vi "Frequency_list_generation.vi"(8 "Type":enum16{"Logarithmic", "Linear"}(ring)=enum."Linear", 9 "Frequency Points":u16=10 min=2 max=10000 step=1, 10 "Stop Frequency (Hz)":u32(slide)=53143 caption="End Frequency (Hz)" scale=30000.0..100000.0, 11 "Start Frequency (Hz)":u32(slide)=53143 scale=30000.0..100000.0) -> (3 "Frequency List":u32[](array[numeric])=[1000, 1002])   [LabVIEW 2018]
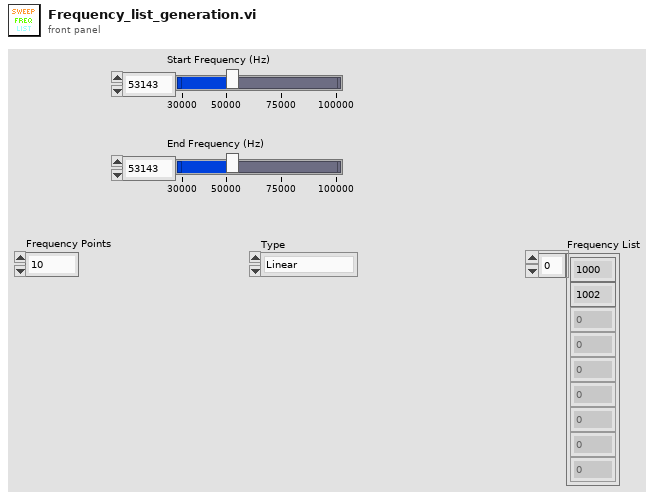
[diagram p1: front panel]
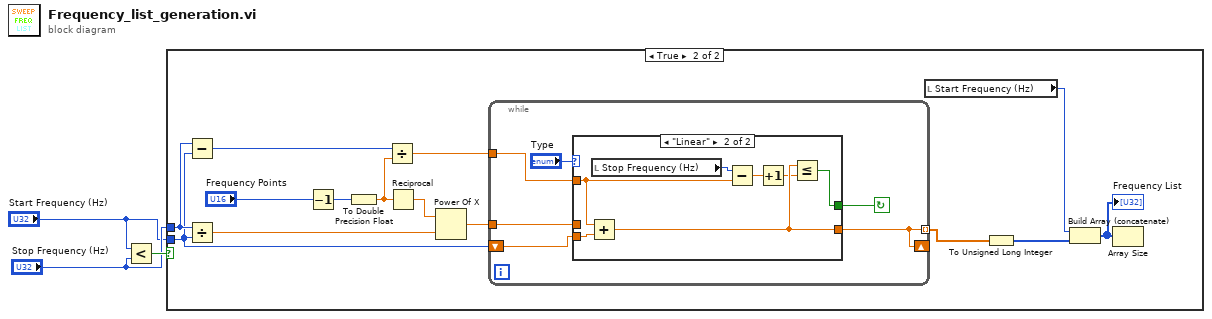
[diagram p0: block diagram]
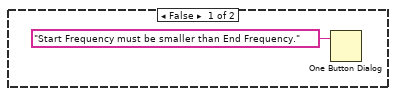
[diagram p2: hidden frame]
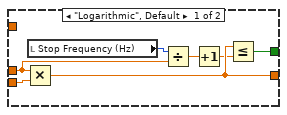
[diagram p3: hidden frame]
diagram:
  n1 = Less?(x="Start Frequency (Hz)", y="Stop Frequency (Hz)") -> (x < y?=w3:bool)
  n2 = case shown="True" w3 {
    tunnel: "Start Frequency (Hz)" -> [_ w13]
    tunnel: "Stop Frequency (Hz)" -> [_ w14]
    frame False {
      n3 = One Button Dialog(message="Start Frequency must be smaller than End Frequency.") -> ()  [unwired: 1 in, 1 out]
    }
    frame True {
      n4 = Subtract(x=w14, y=w13) -> (x-y=w17:u32)
      n5 = Divide(x=w14, y=w13) -> (x/y=w10:dbl)
      n6 = Decrement(x="Frequency Points") -> (x-1=w16:u16)
      n7 = To Double Precision Float(number=w16) -> (double precision float=w12:dbl)
      n8 = Divide(x=w17, y=w12) -> (x/y=w15:dbl)
      n9 = Reciprocal(x=w12) -> (1/x=w11:dbl)
      n10 = Power Of X(1:w10, 2:w11) -> (0:w9:dbl)
      n11 = while {
        shift-right: [w19] -> _
        shift-left: w13 -> [w24]
        tunnel: w15 -> [w22]
        tunnel: w9 -> [w20]
        tunnel: [w19] -> w6 mode=indexing
        stop <- w21 continue-if-true
        n12 = case shown="\"Linear\"" "Type" {
          tunnel: w24 -> [w31 w38]
          tunnel: [w28 w35] -> w19
          tunnel: w22 -> [_ w37]
          tunnel: [w29 w36] -> w21
          tunnel: w20 -> [w30 _]
          frame "Logarithmic", Default {
            n13 = Multiply(x=w30, y=w31) -> (x*y=w28:dbl)
            n14 = local read "Stop Frequency (Hz)"() -> (w25:u32)
            n15 = Divide(x=w25, y=w30) -> (x/y=w27:dbl)
            n16 = Increment(x=w27) -> (x+1=w26:dbl)
            n17 = Less Or Equal?(x=w28, y=w26) -> (x <= y?=w29:bool)
          }
          frame "Linear" {
            n18 = Add(x=w37, y=w38) -> (x+y=w35:dbl)
            n19 = local read "Stop Frequency (Hz)"() -> (w32:u32)
            n20 = Subtract(x=w32, y=w37) -> (x-y=w34:dbl)
            n21 = Increment(x=w34) -> (x+1=w33:dbl)
            n22 = Less Or Equal?(x=w35, y=w33) -> (x <= y?=w36:bool)
          }
        }
      }
      n23 = local read "Start Frequency (Hz)"() -> (w7:u32)
      n24 = To Unsigned Long Integer(number=w6) -> (unsigned 32bit integer=w5:u32[])
      n25 = Build Array (concatenate)(w7, w5) -> (w8:u32[])
      "Frequency List" <- w8
      n26 = Array Size(array=w8) -> ()  [unwired: 1 out]
    }
  }
